vi "Get DIO Bits To Notify Motion Status.vi"(4 "error in (no error)":errorcluster, 6 "Axis (1)":i32=1 min=1 max=3, 7 "VISA resource name":refnum<visa-resource-name>) -> (0 "error out":errorcluster, 1 "Bit Level":bool, 2 "Bit Number":dbl, 3 "VISA resource name out":refnum<visa-resource-name>)   [LabVIEW 2012, in "Newport ESP301.lvlib"]
doc: "Reads the current assignement for notify motion status."
uses:
  Newport ESP301.lvlib
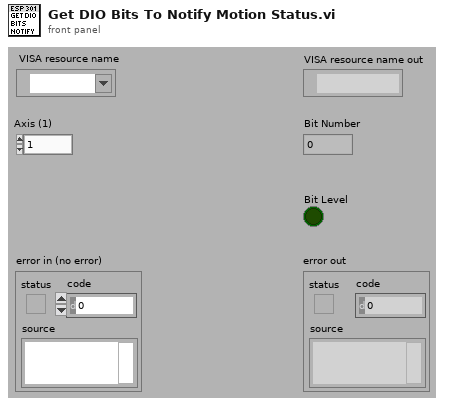
[diagram p1: front panel]
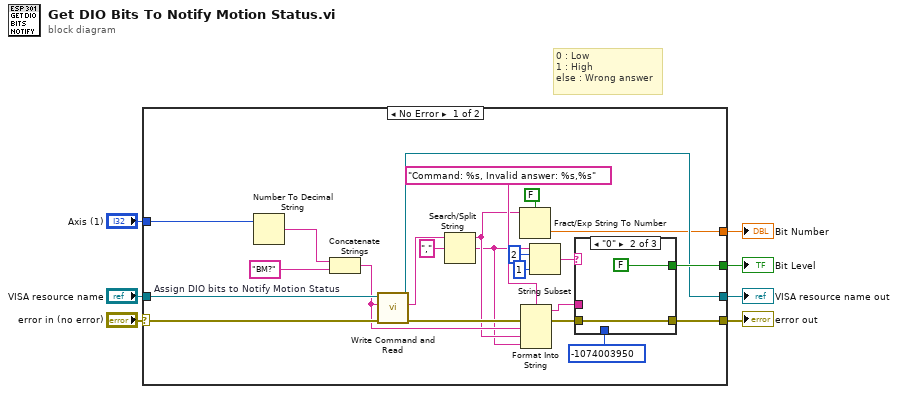
[diagram p0: block diagram]
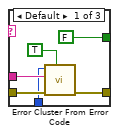
[diagram p2: hidden frame]
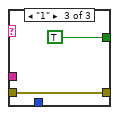
[diagram p3: hidden frame]
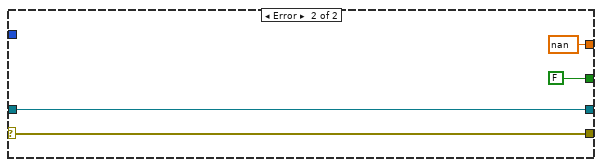
[diagram p4: hidden frame]
diagram:
  # "0 : Low\n1 : High\nelse : Wrong answer"
  n1 = case shown="No Error" "error in (no error)" {
    selector: "error in (no error)" -> [w29 w44]
    tunnel: [w23 w44] -> w7
    tunnel: "VISA resource name" -> [w30 w43]
    tunnel: [w17 w43] -> w6
    tunnel: "Axis (1)" -> [w26 _]
    tunnel: [w22 FALSE ("Motion Done")] -> w2
    tunnel: [w11 nan] -> w1
    frame No Error {
      w27 = "BM?"  # Assign DIO bits to Notify Motion Status
      n2 = Number To Decimal String(number=w26) -> (decimal integer string=w28:string)  [unwired: 1 out]
      n3 = Concatenate Strings(w28, w27) -> (w20:string)
      n4 = call "Write Command and Read.vi"("error in (no error)"=w29, "Command"=w20, "VISA resource name"=w30) -> ("error out"=w25:errorcluster, "Returned string"=w15:string, "VISA resource name out"=w17:refnum<visa-resource-name>)  [unwired: 2 in, 2 out]
      n5 = Search/Split String(string=w15, search string/char (-)=",") -> (substring before match=w10:string, match + rest of string=w9:string)  [unwired: 2 out]
      n6 = Fract/Exp String To Number(use system decimal point (T)=FALSE, string=w10) -> (number=w11:dbl)  [unwired: 3 out]
      n7 = Format Into String(format string="Command: %s, Invalid answer: %s,%s" ("error message (\"\")"), error in=w25, w20, w10, w9) -> (resulting string=w19:string, error out=w24:errorcluster)  [unwired: 1 in]
      n8 = String Subset(string=w9, offset (0)=2, length (rest)=1 ("longueur (reste)")) -> (substring=w21:string)
      n9 = case shown="\"0\"" w21 {
        tunnel: [w35 w37 w39] -> w23
        tunnel: [FALSE ("Motion Done") FALSE ("Motion Done") TRUE ("Motion Done")] -> w22
        tunnel: w24 -> [w33 w37 w39]
        tunnel: w19 -> [w32 _ _]
        tunnel: -1074003950 ("error code (0)") -> [w31 _ _]
        frame Default {
          n10 = call <vilib>:"Error Cluster From Error Code.vi"("show call chain? (False)"=TRUE, "error in (no error)"=w33, "error message (\"\")"=w32, "error code (0)"=w31) -> ("error out"=w35:errorcluster)  [unwired: 5 out]
        }
        frame "0" {
        }
        frame "1" {
        }
      }
    }
    frame Error {
    }
  }
  "error out" <- w7
  "VISA resource name out" <- w6
  "Bit Level" <- w2
  "Bit Number" <- w1
